vi "MathCad_Numeric_Insert_to_Wrkst.vi"(3 "error out 2":errorcluster, 4 "New Variable Name":string, 5 "Mathcad.INumericValue Ref In":refnum<k7>, 6 "Wrksht Ref In":refnum<k7>) -> (0 "error out":errorcluster, 1 "Mathcad.INumericValue Ref Out":refnum<k7>, 2 "Wrksht Ref Out":refnum<k7>)   [LabVIEW 2015]
doc: "Inserts value into the worksheet. This has to be done after the value has been set for the worksheet to recieve the new value."
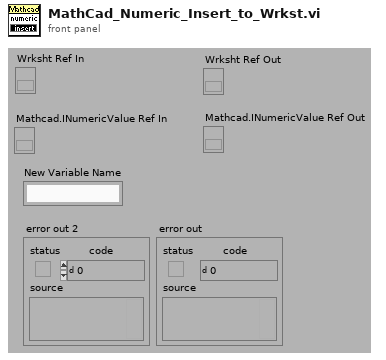
[diagram p1: front panel]
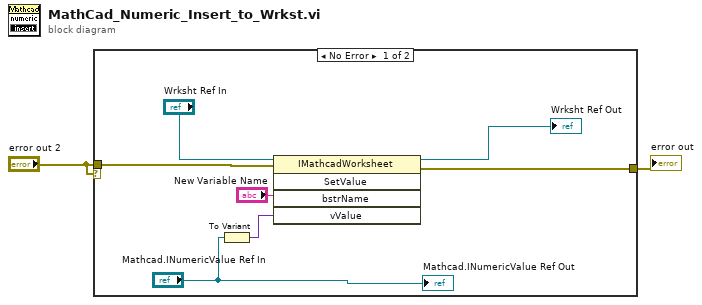
[diagram p0: block diagram]
diagram:
  n1 = case shown="No Error" "error out 2" {
    tunnel: [w9 w10] -> w2
    tunnel: "error out 2" -> [w6 w10]
    frame No Error {
      n2 = To Variant(anything="Mathcad.INumericValue Ref In") -> (Variant=w5:variant)
      n3 = invoke class="IMathcadWorksheet" method="SetValue"(reference="Wrksht Ref In", error in=w6, "bstrName"="New Variable Name", "vValue"=w5) -> (reference out=→"Wrksht Ref Out":refnum<k7>, error out=w9:errorcluster)  [unwired: 1 in, 3 out]
      "Mathcad.INumericValue Ref Out" <- "Mathcad.INumericValue Ref In"
    }
    frame Error {
    }
  }
  "error out" <- w2
